vi "Do.vi"(8 "error in (no error)":errorcluster, 10 "Actor in":refnum<class "Actor.lvclass">, 11 "Display Pop Up Msg Msg":refnum<class "Display Pop Up Msg.lvclass">) -> (0 "error out":errorcluster, 2 "Actor out":refnum<class "Actor.lvclass">)   [LabVIEW 2020, in "Msg.lvlib" / "Display Pop Up Msg.lvclass"]
doc: "This implementation handles the displaying of the Pop Up."
uses:
  Display Pop Up Msg.lvclass
  PPL/HDH.Actor Framework.Core.Actor.lvlibp/1abvi3w/vi.lib/ActorFramework/Actor/Actor.lvclass
  Display Pop Up Msg.lvclass/Display Pop Up Msg.ctl
  Msg.lvlib
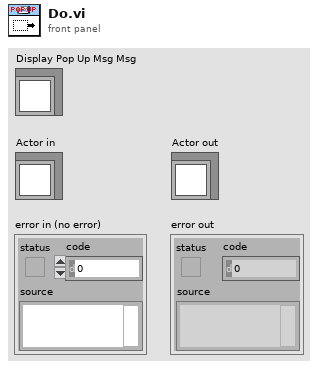
[diagram p1: front panel]
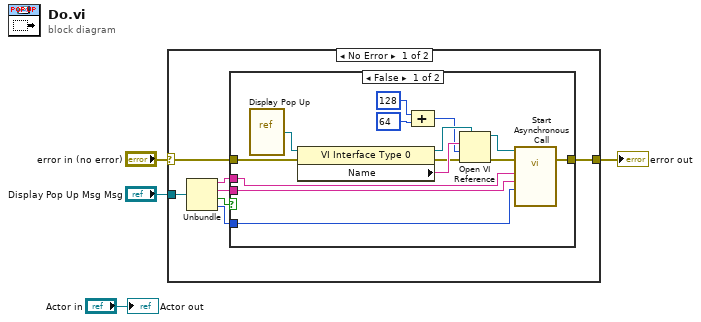
[diagram p0: block diagram]
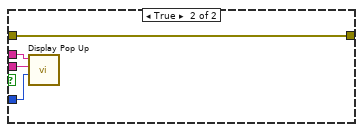
[diagram p2: hidden frame]
diagram:
  n1 = case shown="No Error" "error in (no error)" {
    selector: "error in (no error)" -> [w6 w30]
    tunnel: [w5 w30] -> w2
    tunnel: "Display Pop Up Msg Msg" -> [w11 _]
    frame No Error {
      n2 = Unbundle(w11) -> (w9:string, w8:string, w10:bool, w7:i32)
      n3 = case shown="False" w10 {
        tunnel: w9 -> [w14 w29]
        tunnel: w8 -> [w13 w28]
        tunnel: w7 -> [w12 w27]
        tunnel: w6 -> [w24 w26]
        tunnel: [w15 w26] -> w5
        frame False {
          n4 = vi-ref "Display Pop Up.vi"() -> (w25:refnum<vi>)
          n5 = property class="VI Interface Type 0"(reference=w25, error in=w24) -> (reference out=w23:refnum<vi>, error out=w18:errorcluster, "Name"=w22:string)
          n6 = Compound Arithmetic op=unknown(128 ("options"), 64 ("options")) -> (w20:i32)
          n7 = Open VI Reference(type specifier VI Refnum (for type only)=w23, vi path=w22, options=w20, error in (no error)=w18) -> (vi reference=w17:refnum<vi>, error out=w16:errorcluster)  [unwired: 2 in]
          n8 = call-by-ref "Start Asynchronous Call"(reference=w17, error in=w16, "Pause time out(-1ms)"=w12, "Content"=w13, "Header"=w14) -> (error out=w15:errorcluster)  [unwired: 9 in, 1 out]
        }
        frame True {
          n9 = call "Display Pop Up.vi"("Display time out(-1ms)"=w27, "Content"=w28, "Header"=w29) -> ()  [unwired: 9 in]
        }
      }
    }
    frame Error {
    }
  }
  "error out" <- w2
  "Actor out" <- "Actor in"
